vi "vision_webcam_V1.vi"() -> ()   [LabVIEW 2017]
uses:
  <vilib>/userdefined/High Color/IMAQdx.ctl
  <vilib>/vision/Avi.llb/IMAQ AVI2 Codec Path.ctl
  <vilib>/vision/driver/NI_Vision_Acquisition_Software.lvlib
panel:
  out "Codec Names":string[](array[string])
  in  "stop":bool
  out "Webcam":T1(plugin-control)
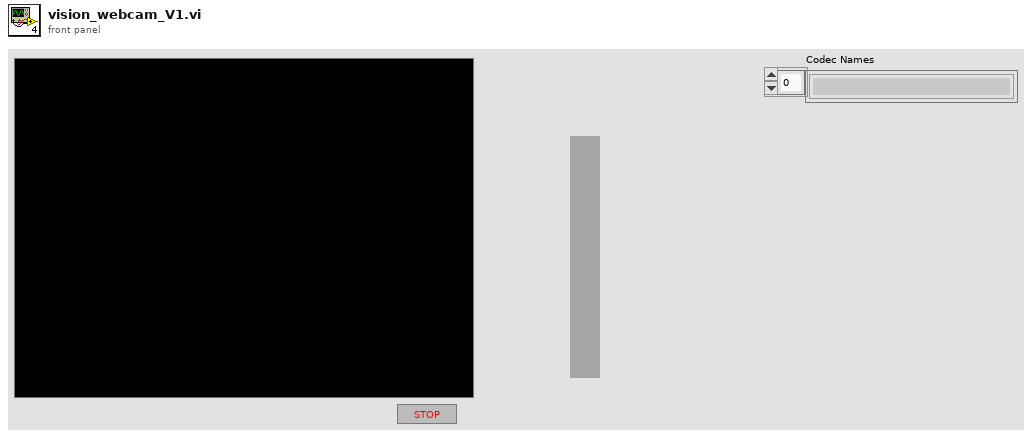
[diagram p1: front panel]
types:
  T1 = typedef "IMAQ Image.ctl" = refnum<image>
  T2 = typedef "IMAQdx.ctl" = refnum<k21>
  T3 = typedef "Image Type" = u32
  T4 = typedef "IMAQ AVI2 Refnum.ctl" = refnum<k20>
  T5 = typedef "IMAQ AVI2 Codec Path.ctl" = u32
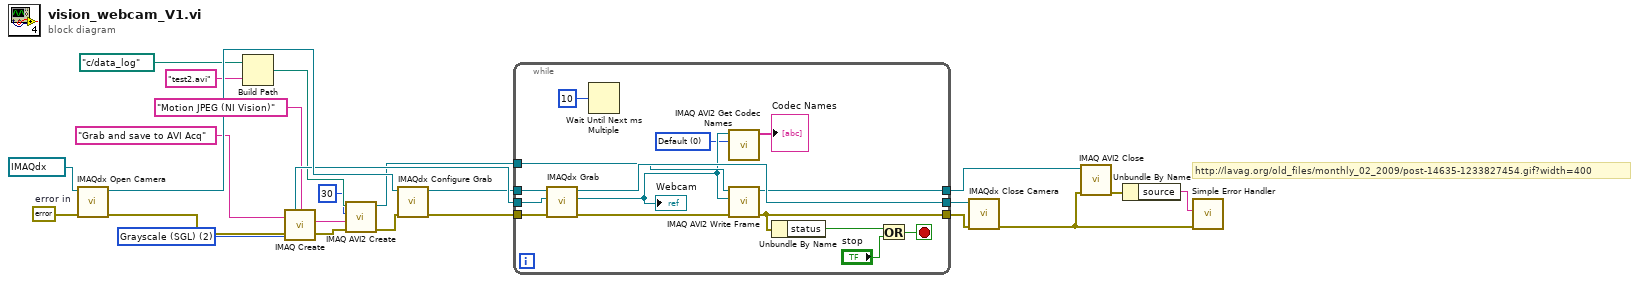
[diagram p0: block diagram]
diagram:
  w6 = T3 2 items=["Grayscale (U8)", "Grayscale (I16)", "Grayscale (SGL)", "Complex (CSG)", "RGB (U32)", "HSL (U32)", "RGB (U64)", "Grayscale (U16)"] ("Image Type")
  w17 = errorcluster {"status"=FALSE, "code"=0, "source"=""}  # error in
  # "http://lavag.org/old_files/monthly_02_2009/post-14635-1233827454.gif?width=400"
  n1 = call <vilib>:"IMAQdx Open Camera.vi"("error in"=w17, "Session In"=T2 "cam0") -> ("error out"=w5:errorcluster, "Session Out"=w23:T2)  [unwired: 8 in]
  n2 = Build Path(base path=path "c:/data_log" ("AVI Path"), name or relative path="test2.avi") -> (appended path=w12:path)
  n3 = call "IMAQ Create"("Image Name"="Grab and save to AVI Acq", "Image Type"=w6, "error in (no error)"=w5) -> ("New Image"=w20:T1, "error out"=w4:errorcluster)  [unwired: 2 in]
  n4 = call "IMAQ AVI2 Create"("error in (no error)"=w4, "Codec"="Motion JPEG (NI Vision)", "Frames Per Second"=u32 30, "AVI Path"=w12) -> ("error out"=w3:errorcluster, "AVI Refnum"=w10:T4)  [unwired: 6 in]
  n5 = call <vilib>:"IMAQdx Configure Grab.vi"("error in"=w3, "Session In"=w23) -> ("error out"=w21:errorcluster, "Session Out"=w2:T2)  [unwired: 8 in]
  n6 = while {
    tunnel: w21 -> [w38]
    tunnel: w2 -> [w37]
    tunnel: w20 -> [w36]
    tunnel: [w30] -> w19
    tunnel: [w35] -> w18
    tunnel: w10 -> [w33]
    tunnel: [w32] -> w7
    stop <- w27 stop-if-true
    w25 = T5 0 items=["Default", "System", "Built in Vision"] ("Codec Source")
    n7 = call <vilib>:"IMAQdx Grab.vi"("error in"=w38, "Image In"=w36, "Session In"=w37) -> ("error out"=w31:errorcluster, "Image Out"=w26:T1, "Session Out"=w35:T2)  [unwired: 5 in, 1 out]
    "Webcam" <- w26
    n8 = Wait Until Next ms Multiple(millisecond multiple=u32 10 ("milliseconds to wait")) -> ()  [unwired: 1 out]
    n9 = call "IMAQ AVI2 Get Codec Names"("Codec Source"=w25, "Image"=w26) -> ("Codec Names"=→"Codec Names":string[])  [unwired: 8 in, 1 out]
    n10 = call "IMAQ AVI2 Write Frame"("error in (no error)"=w31, "Image"=w26, "AVI Refnum"=w33) -> ("error out"=w30:errorcluster, "AVI Refnum (duplicate)"=w32:T4)  [unwired: 6 in, 1 out]
    n11 = Unbundle By Name(w30) -> ("status"=w29:bool)
    n12 = Or(x=w29, y="stop") -> (x .or. y?=w27:bool)
  }
  n13 = call <vilib>:"IMAQdx Close Camera.vi"("error in"=w19, "Session In"=w18) -> ("error out"=w9:errorcluster)  [unwired: 9 in]
  n14 = call "IMAQ AVI2 Close"("error in (no error)"=w9, "AVI Refnum"=w7) -> ("error out"=w8:errorcluster)  [unwired: 9 in]
  n15 = Unbundle By Name(w8) -> ("source"=w15:string)
  n16 = call <vilib>:"Simple Error Handler.vi"("error source (\" \")"=w15, "error in (no error)"=w9) -> ()  [unwired: 3 in, 5 out]
